vi "PT-NMR-ACC-auto.vi"() -> ()   [LabVIEW 2009]
uses:
  <instrlib>/Tektronix TDS 3000 Series/Tektronix TDS 3000 Series.lvlib
panel:
  in  "Seconds to Wait":u32
  in  "Stop Acquisitions":bool
  out "Cumulative Signal":dbl[](graph)
  in  "File name":string
  in  "Comments":string
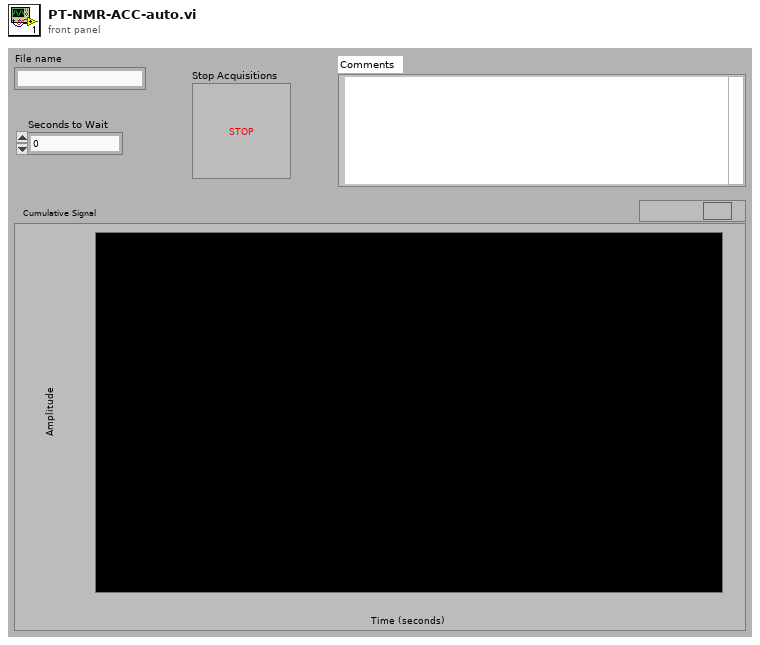
[diagram p1: front panel]
types:
  T1 = enum16{"open", "replace", "create", "open or create", "replace or create", "replace or create with confirmation"}
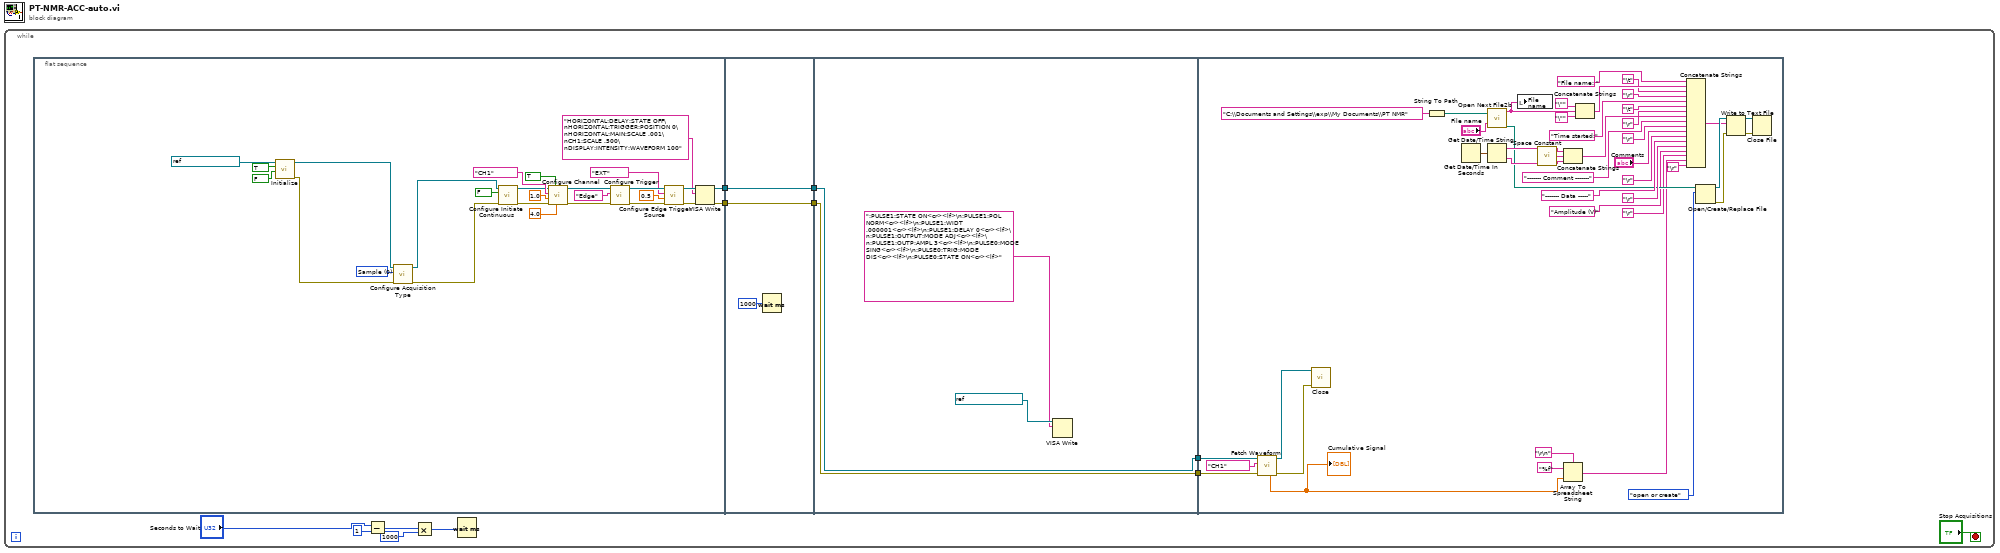
[diagram p0: block diagram]
diagram:
  n1 = while {
    stop <- "Stop Acquisitions" stop-if-true
    n2 = flat-sequence {
      tunnel: [w21] -> w12
      tunnel: [w20] -> w11
      tunnel: w12 -> [w42]
      tunnel: [w42] -> w10
      tunnel: w11 -> [w41]
      tunnel: [w41] -> w9
      tunnel: [w46] -> w8
      tunnel: w10 -> [w46]
      tunnel: [w45] -> w7
      tunnel: w9 -> [w45]
      tunnel: w8 -> [w82]
      tunnel: w7 -> [w81]
      frame #0 {
        w17 = 0 items=["Sample", "Peak Detect", "Envelope", "Average"] ("Acquisition Type (0:Sample)")
        n3 = call <instrlib>:"Initialize.vi"("ID Query (T: Query)"=FALSE, "Reset Device (T: Reset)"=TRUE, "VISA Resource Name"=refnum<visa-resource-name> "GPIB0::3::INSTR" ("VISA resource name")) -> ("error out"=w13:errorcluster, "VISA Resource Name Out"=w14:refnum<visa-resource-name>)  [unwired: 7 in]
        n4 = call <instrlib>:"Configure Acquisition Type.vi"("error in (no error)"=w13, "Acquisition Type (0:Sample)"=w17, "VISA Resource Name"=w14) -> ("error out"=w15:errorcluster, "VISA Resource Name Out"=w16:refnum<visa-resource-name>)  [unwired: 7 in]
        n5 = call <instrlib>:"Configure Initiate Continuous.vi"("error in (no error)"=w15, "Continuous Acquisition (False)"=FALSE, "VISA Resource Name"=w16) -> ("error out"=w24:errorcluster, "VISA Resource Name Out"=w25:refnum<visa-resource-name>)  [unwired: 7 in]
        n6 = call <instrlib>:"Configure Channel.vi"("Vertical Range (10.0 V)"=4.0, "Channel Enabled (True)"=TRUE, "error in (no error)"=w24, "Probe Attenuation (1.0)"=1.0, "Channel Name (\"CH1\")"="CH1" ("Channel Name (\"CH1\")"), "VISA Resource Name"=w25) -> ("error out"=w33:errorcluster, "VISA Resource Name Out"=w35:refnum<visa-resource-name>)  [unwired: 4 in]
        n7 = call <instrlib>:"Configure Trigger.vi"("error in (no error)"=w33, "Trigger Type (Edge)"="Edge", "VISA Resource Name"=w35) -> ("error out"=w31:errorcluster, "VISA Resource Name Out"=w32:refnum<visa-resource-name>)  [unwired: 7 in]
        n8 = call <instrlib>:"Configure Edge Trigger Source.vi"("error in (no error)"=w31, "Trigger Level (0.0 V)"=0.5, "Trigger Source (Channel 1)"="EXT", "VISA Resource Name"=w32) -> ("error out"=w23:errorcluster, "VISA Resource Name Out"=w22:refnum<visa-resource-name>)  [unwired: 6 in]
        n9 = VISA Write(VISA resource name=w22, write buffer="HORIZONTAL:DELAY:STATE OFF\nHORIZONTAL:TRIGGER:POSITION 0\nHORIZONTAL:MAIN:SCALE .001\nCH1:SCALE .500\nDISPLAY:INTENSITY:WAVEFORM 100", error in (no error)=w23) -> (VISA resource name out=w21:refnum<visa-resource-name>, error out=w20:errorcluster)  [unwired: 1 out]
      }
      frame #1 {
        n10 = Wait (ms)(milliseconds to wait=u32 1000) -> ()  [unwired: 1 out]
      }
      frame #2 {
        n11 = VISA Write(VISA resource name=refnum<visa-resource-name> "GPIB0::7::INSTR", write buffer=":PULSE1:STATE ON<cr><lf>\n:PULSE1:POL NORM<cr><lf>\n:PULSE1:WIDT .000001<cr><lf>\n:PULSE1:DELAY 0<cr><lf>\n:PULSE1:OUTPUT:MODE ADJ<cr><lf>\n:PULSE1:OUTP:AMPL 3<cr><lf>\n:PULSE0:MODE SING<cr><lf>\n:PULSE0:TRIG:MODE DIS<cr><lf>\n:PULSE0:STATE ON<cr><lf>") -> ()  [unwired: 1 in, 3 out]
      }
      frame #3 {
        n12 = call <instrlib>:"Fetch Waveform.vi"("error in (no error)"=w81, "Source (Channel 1)"="CH1", "VISA Resource Name"=w82) -> ("error out"=w47:errorcluster, "VISA Resource Name Out"=w48:refnum<visa-resource-name>, "Waveform Array"=w80:dbl[])  [unwired: 3 in, 3 out]
        "Cumulative Signal" <- w80
        n13 = call <instrlib>:"Close.vi"("error in (no error)"=w47, "VISA Resource Name"=w48) -> ()  [unwired: 9 in, 1 out]
        n14 = String To Path(string="C:\\Documents and Settings\\exp\\My Documents\\PT NMR" ("format string")) -> (path=w57:path)
        n15 = Get Date/Time In Seconds() -> (seconds since 1Jan1904=w70:timestamp)
        n16 = call "Open Next File2b.vi"("Input File Pattern"="File name", "Dir Path"=w57) -> ("appended path"=w56:path, "Output File Name"=w54:string)  [unwired: 2 in, 1 out]
        n17 = Get Date/Time String(seconds (now)=w70) -> (date string=w69:string, time string=w67:string)  [unwired: 2 in]
        n18 = local write "File name"(w54) -> ()
        n19 = call <vilib>:"Space Constant.vi"() -> ("String"=w68:string)
        n20 = Concatenate Strings(w69, w68, w67) -> (w66:string)
        n21 = Array To Spreadsheet String(delimiter (Tab)="\r\n", array=w80, 3:"%f" ("format string")) -> (spreadsheet string=w49:string)
        n22 = Concatenate Strings("\"" ("string"), w54, "\"" ("string")) -> (w72:string)
        n23 = Concatenate Strings("File name: " ("string"), "\t", w72, "\r", "Time started:" ("string"), "\t", w66, "\r" ("string"), "------- Comment -------" ("string"), "\r" ("string"), "Comments", "\r", "------- Data -----" ("string"), "\r", "Amplitude (V)", "\r", w49, "\r") -> (w53:string)
        n24 = Open/Create/Replace File(file path (use dialog)=w56, operation (0:open)=T1."open or create") -> (refnum out=w89:refnum<file>, error out=w87:errorcluster)  [unwired: 4 in, 1 out]
        n25 = Write to Text File(file (use dialog)=w89, text=w53, error in=w87) -> (refnum out=w88:refnum<file>, error out=w86:errorcluster)  [unwired: 1 in, 1 out]
        n26 = Close File(refnum=w88, error in=w86) -> ()  [unwired: 2 out]
      }
    }
    n27 = Subtract(x="Seconds to Wait", y=u32 1) -> (x-y=w2:u32)
    n28 = Multiply(x=w2, y=u32 1000) -> (x*y=w1:u32)
    n29 = Wait (ms)(milliseconds to wait=w1) -> ()  [unwired: 1 out]
  }
